vi "Next or Error.vi"(4 "error in (no error)":errorcluster, 7 "State in":T1) -> (3 "State out":T1)   [LabVIEW 2014, in "Startup Processes.lvlib"]
uses:
  Startup Processes.lvlib
  _typedefs/States.ctl
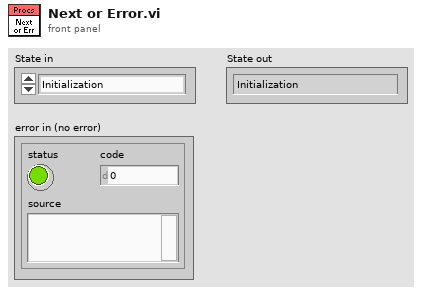
[diagram p1: front panel]
types:
  T1 = typedef "Startup Processes.lvlib/States.ctl" = enum16{"Initialization", "Read Input", "Test Fan Limits", "Set Fan", "Test Cooler Limits", "Set Cooler", "Acquisition TO Wait", "Error", "Deinitialize"}
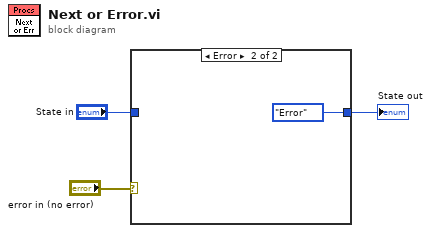
[diagram p0: block diagram]
diagram:
  n1 = case shown="Error" "error in (no error)" {
    tunnel: [w4 States."Error" ("State in")] -> w2
    tunnel: "State in" -> [w4 _]
    frame No Error {
    }
    frame Error {
    }
  }
  "State out" <- w2
